vi "Reset Sim.vi"(8 "error in (no error)":errorcluster, 11 "FPGA Sim in":refnum<class "FPGA Sim.lvclass">) -> (0 "error out":errorcluster, 3 "FPGA Sim out":refnum<class "FPGA Sim.lvclass">)   [LabVIEW 2020, in "Unit Tests.lvlib" / "FPGA Sim.lvclass"]
uses:
  FPGA Sim.lvclass
  FPGA Sim.lvclass/FPGA Sim.ctl
  Dependencies/Virtual Memory Unit/Virtual Memory Unit.lvclass
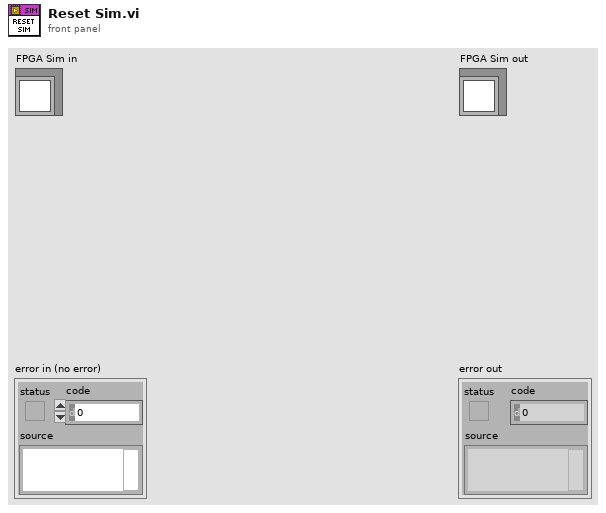
[diagram p1: front panel]
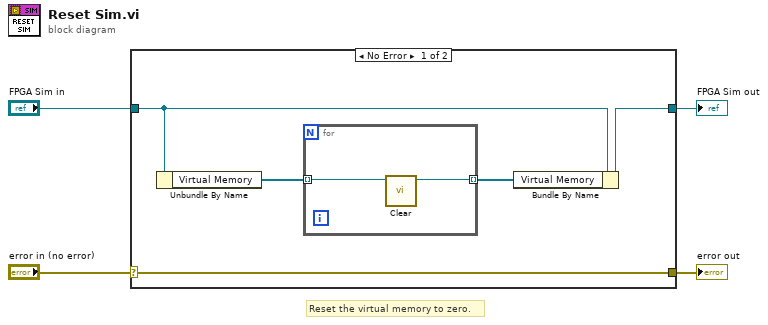
[diagram p0: block diagram]
diagram:
  # "Reset the virtual memory to zero."
  n1 = case shown="No Error" "error in (no error)" {
    selector: "error in (no error)" -> [w9 w13]
    tunnel: [w9 w13] -> w3
    tunnel: [w7 w12] -> w1
    tunnel: "FPGA Sim in" -> [w8 w12]
    frame No Error {
      n2 = Unbundle By Name(w8) -> ("Virtual Memory"=w6:refnum<class "Virtual Memory Unit.lvclass">[])
      n3 = for {
        tunnel: w6 -> [w11] mode=indexing
        tunnel: [w10] -> w5 mode=indexing
        n4 = call "Clear.vi"("Virtual Memory Unit in"=w11) -> ("Virtual Memory Unit out"=w10:refnum<class "Virtual Memory Unit.lvclass">)  [unwired: 9 in, 1 out]
      }
      n5 = Bundle By Name(cluster=w8, "Virtual Memory"=w5) -> (w7:refnum<class "FPGA Sim.lvclass">)
    }
    frame Error {
    }
  }
  "error out" <- w3
  "FPGA Sim out" <- w1
